vi "Set XY Acceleration.vi"(8 "error in (no error)":errorcluster, 10 "mm/s":dbl=200.0 format="%#_13g", 11 "Gantry 2":refnum<k24>) -> (0 "error out":errorcluster, 2 "Array":dbl[](array[numeric]), 3 "Gantry 3":refnum<k24>)   [LabVIEW 2020, in "A3200.lvclass"]
uses:
  A3200.lvclass
  C:/Program Files (x86)/Aerotech/A3200/LabVIEW/2010/Bin/Aerotech.A3200.dll
  Program Files (x86)/Aerotech/A3200/LabVIEW/2010/Bin/Aerotech.A3200.dll
  Aerotech.lvlib
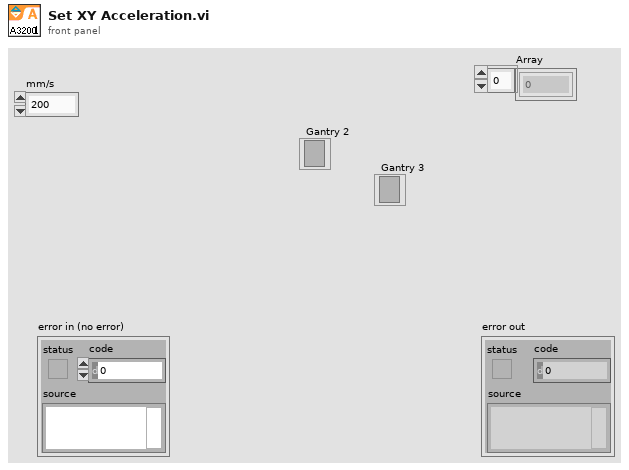
[diagram p1: front panel]
types:
  T1 = cluster{"Status":bool, "Error Code":i32, "Source":string}
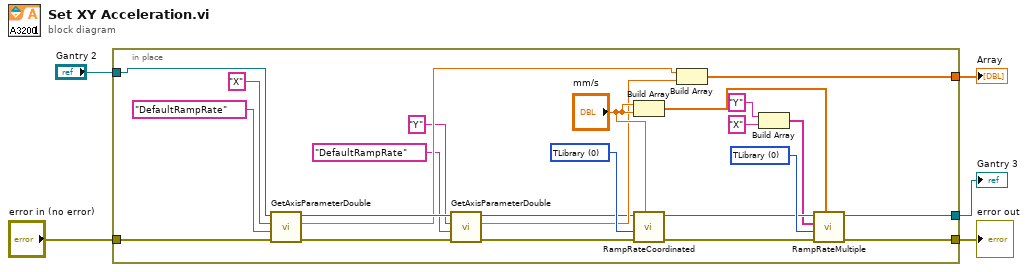
[diagram p0: block diagram]
diagram:
  n1 = in-place {
    in-place-border: "Gantry 2" -> [w17]
    in-place-border: [w21] -> w1
    in-place-border: [w20] -> w5
    in-place-border: "error in (no error)" -> [w14]
    in-place-border: [w18] -> w3
    w27 = 0 items=["TLibrary", "T01", "T02", "T03", "T04", "T05", "T06", "T07", "T08", "T09", "T10", "T11", "T12", "T13", "T14", "T15", "T16", "T17", "T18", "T19", "T20", "T21", "T22", "T23", "T24", "T25", "T26", "T27", "T28", "T29", "T30", "T31"] ("task id")
    w28 = 0 items=["TLibrary", "T01", "T02", "T03", "T04", "T05", "T06", "T07", "T08", "T09", "T10", "T11", "T12", "T13", "T14", "T15", "T16", "T17", "T18", "T19", "T20", "T21", "T22", "T23", "T24", "T25", "T26", "T27", "T28", "T29", "T30", "T31"] ("taskId")
    n2 = call "GetAxisParameterDouble.vi"("error in (no error)"=w14, "Parameter Name"="DefaultRampRate", "axis name"="X", "controller in"=w17) -> ("error out"=w11:errorcluster, "value"=w12:dbl, "controller out"=w13:refnum<k24>)  [unwired: 5 in]
    n3 = call "GetAxisParameterDouble.vi"("error in (no error)"=w11, "Parameter Name"="DefaultRampRate", "axis name"="Y", "controller in"=w13) -> ("error out"=w10:errorcluster, "value"=w9:dbl, "controller out"=w8:refnum<k24>)  [unwired: 5 in]
    n4 = Build Array("mm/s", "mm/s") -> (w29:dbl[])
    n5 = call "RampRateCoordinated.vi"("ramp rate"="mm/s", "error in (no error)"=w10, "taskId"=w28, "controller in"=w8) -> ("error out"=w19:T1, "controller out"=w26:refnum<k24>)  [unwired: 6 in]
    n6 = Build Array(w12, w9) -> (w20:dbl[])
    n7 = Build Array("Y", "X") -> (w23:string[])
    n8 = call "RampRateMultiple.vi"("ramp rates"=w29, "error in (no error)"=w19, "task id"=w27, "axis names"=w23, "controller in"=w26) -> ("error out (no error)"=w18:T1, "controller out"=w21:refnum<k24>)  [unwired: 5 in]
  }
  "error out" <- w3
  "Array" <- w5
  "Gantry 3" <- w1
